vi "initAO_Tasks.vi"(5 "maximum value":dbl=10.0, 7 "minimum value":dbl=-10.0, 8 "error in (no error)":errorcluster, 11 "DAQmx Device Name 2":tag="Dev2") -> (0 "error out":errorcluster, 1 "DI tasks":refnum<k21>, 2 "DO tasks":refnum<k21>, 3 "AO tasks":refnum<k21>)   [LabVIEW 2011]
uses:
  OnOffTypeDef.ctl
  C:/Program Files/National Instruments/LabVIEW 2011/resource/objmgr/daqmx.rc
panel:
  out "DI.Ports":tag[](array[tag])
  out "DO.Lines":tag[](array[tag])
  out "Numeric":i32
  out "Channels":refnum<k21>[](array[refnum])
  out "AO.PhysicalChans":tag[](array[tag])
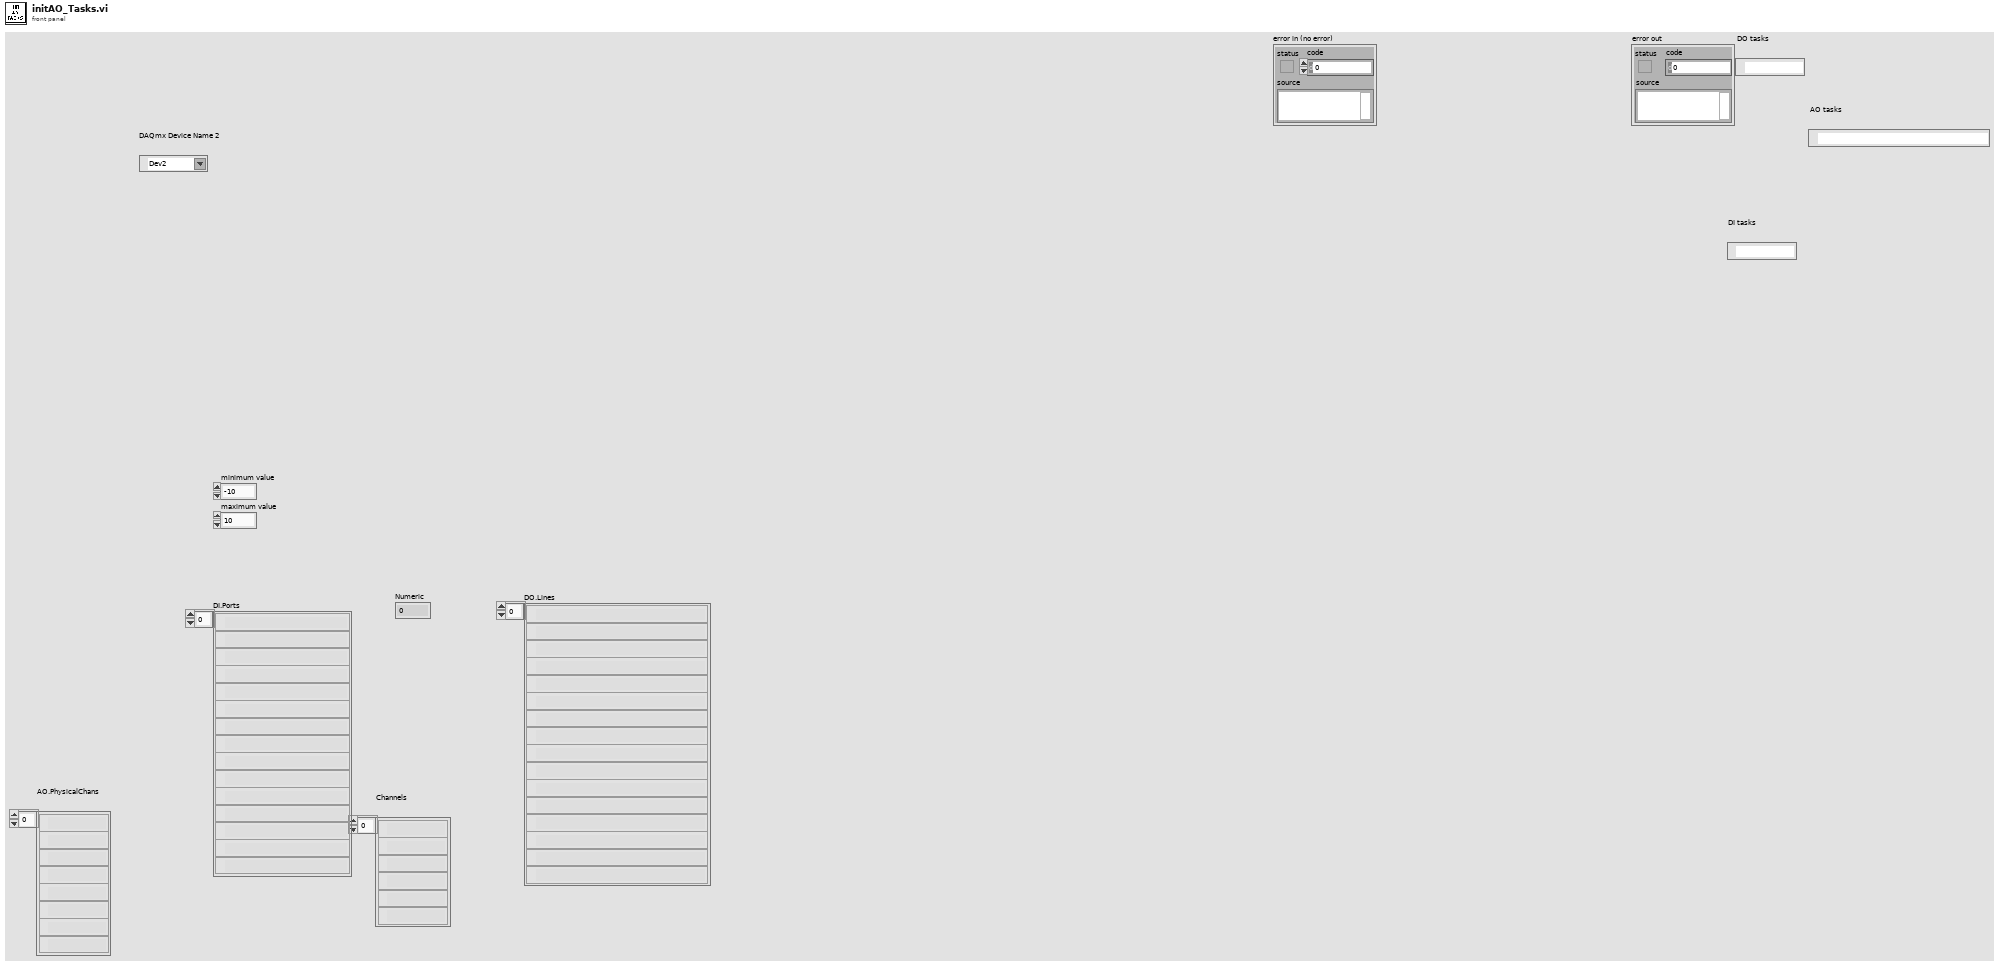
[diagram p1: front panel]
types:
  T1 = typedef "OnOffTypeDef.ctl" = enum16{"off", "on"}
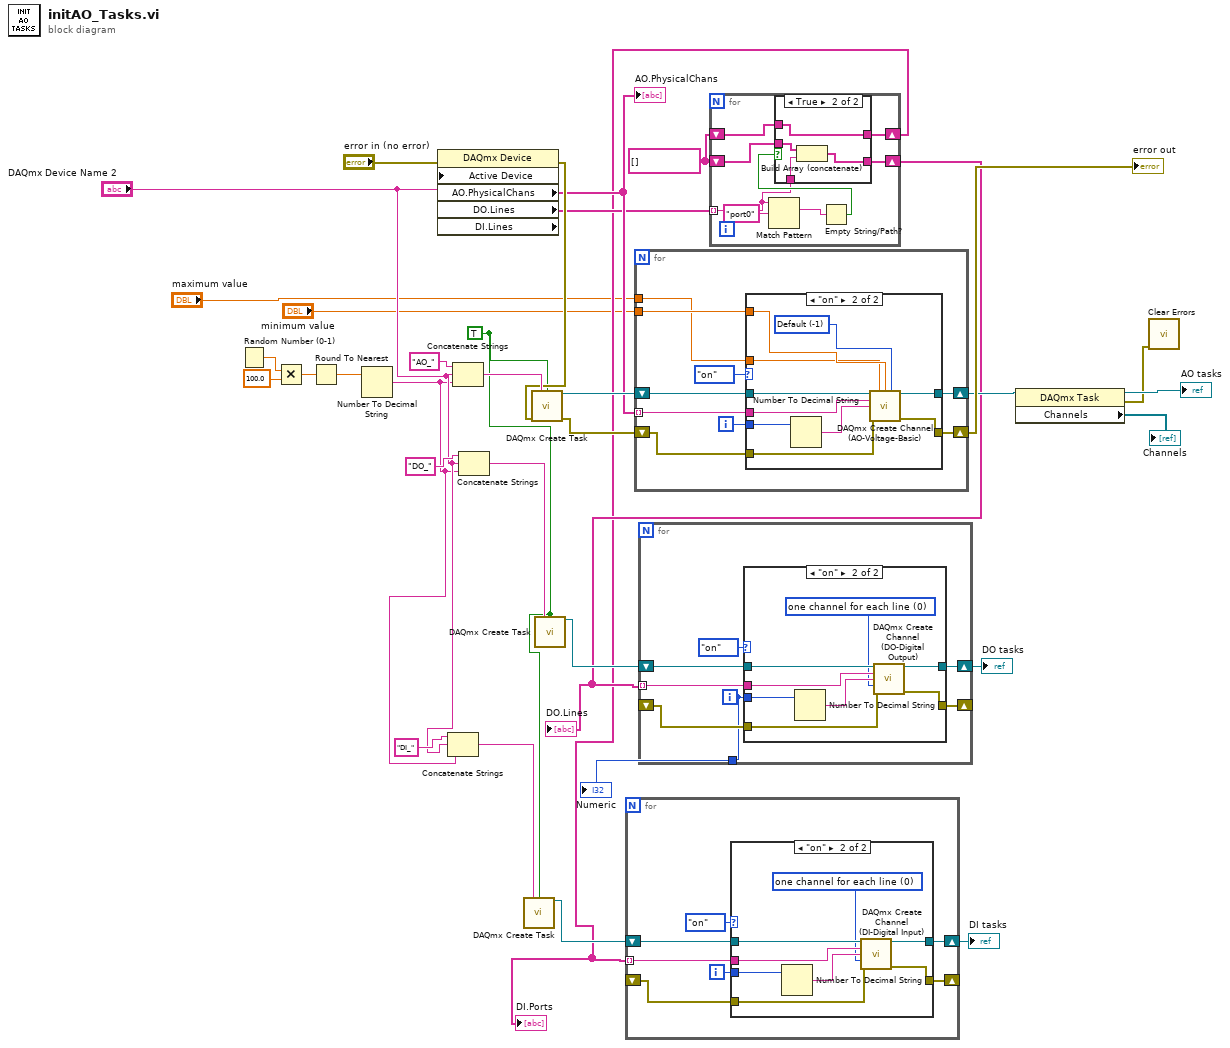
[diagram p0: block diagram]
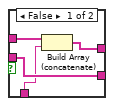
[diagram p2: hidden frame]
diagram:
  w5 = tag[] []
  w13 = TRUE ("auto cleanup")
  n1 = Random Number (0-1)() -> (number: 0 to 1=w31:dbl)
  n2 = Multiply(x=w31, y=100.0) -> (x*y=w33:dbl)
  n3 = Round To Nearest(number=w33) -> (nearest integer value=w34:dbl)
  n4 = Number To Decimal String(number=w34) -> (decimal integer string=w15:string)  [unwired: 1 in]
  n5 = property class="DAQmx Device" props=["Active Device", "AO.PhysicalChans", "DO.Lines", "DI.Lines"](error in="error in (no error)", "Active Device"="DAQmx Device Name 2") -> (error out=w26:errorcluster, "AO.PhysicalChans"=w9:tag[], "DO.Lines"=w6:tag[])  [unwired: 1 in, 2 out]
  "AO.PhysicalChans" <- w9
  n6 = Concatenate Strings("DI_", "DAQmx Device Name 2", w15) -> (w18:string)
  n7 = Concatenate Strings("AO_", "DAQmx Device Name 2", w15) -> (w29:string)
  n8 = Concatenate Strings("DO_", "DAQmx Device Name 2", w15) -> (w22:string)
  n9 = call "DAQmx Create Task.vi"("new task name"=w18, "auto cleanup"=w13) -> ("task out"=w14:refnum<k21>)  [unwired: 12 in, 1 out]
  n10 = call "DAQmx Create Task.vi"("new task name"=w29, "auto cleanup"=w13, "error in"=w26) -> ("task out"=w28:refnum<k21>, "error out"=w25:errorcluster)  [unwired: 11 in]
  n11 = call "DAQmx Create Task.vi"("new task name"=w22, "auto cleanup"=w13) -> ("task out"=w21:refnum<k21>)  [unwired: 12 in, 1 out]
  n12 = for {
    tunnel: w9 -> [w40] mode=indexing
    shift-right: [w41] -> w12
    shift-left: w28 -> [w43]
    shift-right: [w37] -> w24
    shift-left: w25 -> [w38]
    tunnel: "minimum value" -> [w36]
    tunnel: "maximum value" -> [w35]
    i -> [w42]
    n13 = case shown="\"on\"" OnOffTypeDef."on" ("Channel 0") {
      tunnel: w43 -> [w45 w55]
      tunnel: w42 -> [_ w54]
      tunnel: [w45 w52] -> w41
      tunnel: w40 -> [_ w51]
      tunnel: w38 -> [w44 w49]
      tunnel: [w44 w48] -> w37
      tunnel: w36 -> [_ w47]
      tunnel: w35 -> [_ w46]
      frame "off", Default {
      }
      frame "on" {
        w50 = -1 items=["Default"=-1, "RSE"=10083, "Differential"=10106, "Pseudodifferential"=12529] ("output terminal configuration")
        n14 = Number To Decimal String(number=w54) -> (decimal integer string=w53:string)  [unwired: 1 in]
        n15 = call "DAQmx Create Channel (AO-Voltage-Basic).vi"("task in"=w55, "maximum value"=w46, "minimum value"=w47, "output terminal configuration"=w50, "physical channels"=w51, "name to assign"=w53, "error in"=w49) -> ("task out"=w52:refnum<k21>, "error out"=w48:errorcluster)  [unwired: 7 in]
      }
    }
  }
  "error out" <- w24
  n16 = for {
    tunnel: w6 -> [w60] mode=indexing
    shift-right: [w56] -> w3
    shift-left: w5 -> [w57]
    shift-right: [w59] -> w4
    shift-left: w5 -> [w58]
    n17 = Match Pattern(string=w60, regular expression="port0") -> (match substring=w62:string)  [unwired: 1 in, 3 out]
    n18 = Empty String/Path?(string/path=w62) -> (empty?=w61:bool)
    n19 = case shown="True" w61 {
      tunnel: w60 -> [w66 w71]
      tunnel: [w67 w70] -> w59
      tunnel: w58 -> [w67 w69]
      tunnel: [w65 w68] -> w56
      tunnel: w57 -> [w64 w68]
      frame False {
        n20 = Build Array (concatenate)(w64, w66) -> (w65:tag[])
      }
      frame True {
        n21 = Build Array (concatenate)(w69, w71) -> (w70:tag[])
      }
    }
  }
  "DO.Lines" <- w4
  "DI.Ports" <- w3
  n22 = for {
    tunnel: w3 -> [w75] mode=indexing
    shift-right: [w76] -> w19
    shift-left: w14 -> [w78]
    shift-right: [w72] -> _
    shift-left: _ -> [w73]
    i -> [w77]
    n23 = case shown="\"on\"" OnOffTypeDef."on" ("Channel 0") {
      tunnel: w78 -> [w80 w88]
      tunnel: w77 -> [_ w87]
      tunnel: [w80 w85] -> w76
      tunnel: w75 -> [_ w84]
      tunnel: w73 -> [w79 w83]
      tunnel: [w79 w82] -> w72
      frame "off", Default {
      }
      frame "on" {
        w81 = 0 items=["one channel for each line", "one channel for all lines"] ("line grouping")
        n24 = Number To Decimal String(number=w87) -> (decimal integer string=w86:string)  [unwired: 1 in]
        n25 = call "DAQmx Create Channel (DI-Digital Input).vi"("task in"=w88, "lines"=w84, "name to assign"=w86, "line grouping"=w81, "error in"=w83) -> ("task out"=w85:refnum<k21>, "error out"=w82:errorcluster)  [unwired: 9 in]
      }
    }
  }
  "DI tasks" <- w19
  n26 = for {
    tunnel: w4 -> [w93] mode=indexing
    shift-right: [w94] -> w20
    shift-left: w21 -> [w95]
    shift-right: [w90] -> _
    shift-left: _ -> [w91]
    tunnel: [w89] -> w7
    i -> [w89]
    n27 = case shown="\"on\"" OnOffTypeDef."on" ("Channel 0") {
      tunnel: w95 -> [w97 w105]
      tunnel: w89 -> [_ w104]
      tunnel: [w97 w102] -> w94
      tunnel: w93 -> [_ w101]
      tunnel: w91 -> [w96 w100]
      tunnel: [w96 w99] -> w90
      frame "off", Default {
      }
      frame "on" {
        w98 = 0 items=["one channel for each line", "one channel for all lines"] ("line grouping")
        n28 = Number To Decimal String(number=w104) -> (decimal integer string=w103:string)  [unwired: 1 in]
        n29 = call "DAQmx Create Channel (DO-Digital Output).vi"("task in"=w105, "lines"=w101, "name to assign"=w103, "line grouping"=w98, "error in"=w100) -> ("task out"=w102:refnum<k21>, "error out"=w99:errorcluster)  [unwired: 9 in]
      }
    }
  }
  "DO tasks" <- w20
  "Numeric" <- w7
  n30 = property class="DAQmx Task"(reference=w12) -> (reference out=→"AO tasks":refnum<k21>, error out=w10:errorcluster, "Channels"=→"Channels":refnum<k21>[])  [unwired: 1 in]
  n31 = call "Clear Errors.vi"("error in (no error)"=w10) -> ()  [unwired: 6 in, 1 out]
